vi "Result_Test.vi"(8 "error in (no error)":errorcluster caption="entrée d'erreur (pas d'erreur)", 11 "Get_Voltage en entrée":refnum<class "Read_HUE_LED.lvclass">) -> (0 "error out":errorcluster caption="sortie d'erreur", 3 "Get_Voltage en sortie":refnum<class "Read_HUE_LED.lvclass">)   [LabVIEW 2020, in "Library Test.lvlib" / "Read_HUE_LED.lvclass"]
uses:
  Read_HUE_LED.lvclass
  C:/Users/ngarcin/OneDrive - Altyor/Standard TB/Class/Test/Test (Default)/Test (Default).lvclass
  JSON API/JSON Value/Set from JSON string.vi
  Instrument/Instrument (Default)/Class Instrument (Default).lvclass
  JSON API/JSON Value/JSON Value.lvclass
  Read_Led_Analyser/Read_Led_Analyser.lvclass
  Read_HUE_LED.lvclass/Read_HUE_LED.ctl
  JSON API/Variant JSON/Variant JSON.lvlib
  JSON API/Get Polymorphic/JSON GetSet.lvlib
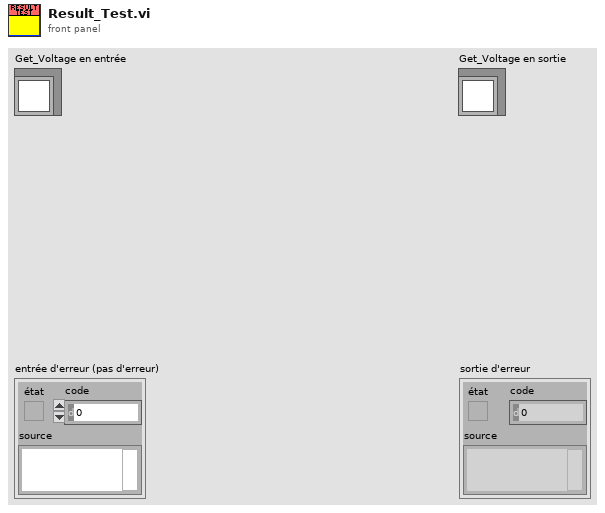
[diagram p1: front panel]
types:
  T1 = cluster{"Hue":dbl, "Saturation":u32, "Intensity":u32}
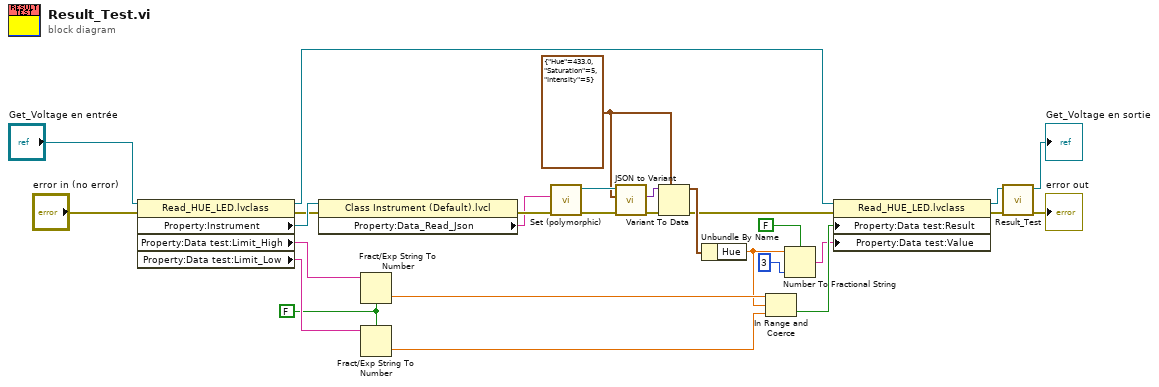
[diagram p0: block diagram]
diagram:
  w1 = FALSE ("utiliser le séparateur décimal du système (V)")
  w20 = T1 {"Hue"=433.0, "Saturation"=5, "Intensity"=5} ("Parameter")
  n1 = property class="Read_HUE_LED.lvclass"(reference="Get_Voltage en entrée", error in="error in (no error)") -> (reference out=w17:refnum<class "Read_HUE_LED.lvclass">, error out=w5:errorcluster, "Property:Instrument"=w6:refnum<class "Class Instrument (Default).lvclass">, "Property:Data test:Limit_High"=w15:string, "Property:Data test:Limit_Low"=w14:string)
  n2 = property class="Class Instrument (Default).lvcl"(reference=w6, error in=w5) -> (error out=w4:errorcluster, "Property:Data_Read_Json"=w3:string)  [unwired: 1 out]
  n3 = Fract/Exp String To Number(use system decimal point (T)=w1, string=w15) -> (number=w13:dbl)  [unwired: 2 in, 1 out]
  n4 = Fract/Exp String To Number(use system decimal point (T)=w1, string=w14) -> (number=w12:dbl)  [unwired: 2 in, 1 out]
  n5 = call-poly "Set (polymorphic).vi"("error in (no error)"=w4, "JSON stream"=w3) -> ("error out"=w24:errorcluster, "JSON Value out"=w22:refnum<class "JSON Value.lvclass">)  [unwired: 7 in, 1 out]
  n6 = call "JSON to Variant.vi"("error in (no error)"=w24, "Variant (Data Type)"=w20, "JSON Value"=w22) -> ("error out"=w23:errorcluster, "Variant out"=w21:variant)  [unwired: 7 in]
  n7 = Variant To Data(error in=w23, type=w20, Variant=w21) -> (data=w19:T1, error out=w7:errorcluster)
  n8 = Unbundle By Name(w19) -> ("Hue"=w10:dbl)
  n9 = In Range and Coerce(upper limit=w13, x=w10, lower limit=w12) -> (In Range?=w11:bool)  [unwired: 1 out]
  n10 = Number To Fractional String(use system decimal point (T)=FALSE ("utiliser le séparateur décimal du système (V)"), number=w10, precision (6)=i16 3 ("précision (6)")) -> (F-format string=w9:string)  [unwired: 1 in]
  n11 = property class="Read_HUE_LED.lvclass"(reference=w17, error in=w7, "Property:Data test:Result"=w11, "Property:Data test:Value"=w9) -> (reference out=w16:refnum<class "Read_HUE_LED.lvclass">, error out=w18:errorcluster)
  n12 = call-parent "Result_Test.vi"("error in (no error)"=w18, "Get_Voltage en entrée"=w16) -> ("error out"=→"error out":errorcluster, "Get_Voltage en sortie"=→"Get_Voltage en sortie":refnum<class "Read_HUE_LED.lvclass">)  [unwired: 8 in]
